vi "randclur.vi"   [LabVIEW 2020]
uses:
  <vilib>/numeric/Random Number (Range) U64.vi
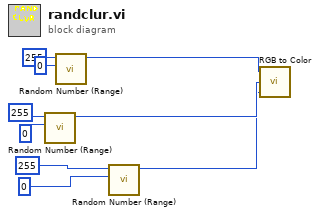
[diagram p0: block diagram]
diagram:
  n1 = call-poly <vilib>:"Random Number (Range).vi"("lower bound (0)"=u64 0, "upper bound (100)"=u64 255) -> ("number"=w8:u64)  [unwired: 9 in]
  n2 = call-poly <vilib>:"Random Number (Range).vi"("lower bound (0)"=u64 0, "upper bound (100)"=u64 255) -> ("number"=w9:u64)  [unwired: 9 in]
  n3 = call-poly <vilib>:"Random Number (Range).vi"("lower bound (0)"=u64 0, "upper bound (100)"=u64 255) -> ("number"=w7:u64)  [unwired: 9 in]
  n4 = call <vilib>:"RGB to Color.vi"("B"=w7, "G"=w8, "R"=w9) -> ()  [unwired: 1 out]
